vi "NI VeriStand - Get Item Property.vi"   [LabVIEW 2020, in "Custom Device API.lvlib"]
doc: "Returns the <B>Value</B> of a specific item <B>Property Name</B>. Properties do not inherit within a custom device, so <B>Item Ref in</B> must reference the specific item on which the property is set. \n\nFor instances with a <B>Default Value</B> input, the <B>Value</B> output returns this value if the <B>Property Name</B> is not found for the specified item. Wire data to the <B>Default Value</B> input to determine the polymorphic instance to use or manually select the instance."
uses:
  <vilib>/NI VeriStand/Custom Device API/Custom Device API.lvlib
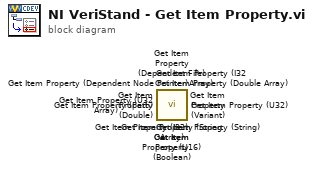
[diagram p0: block diagram]
diagram:
  n1 = call <vilib>:"Get Item Property (String Array).vi"() -> ()  [unwired: 8 in, 4 out]
  n2 = call <vilib>:"Get Item Property (I32 Array).vi"() -> ()  [unwired: 8 in, 4 out]
  n3 = call <vilib>:"Get Item Property (U32 Array).vi"() -> ()  [unwired: 8 in, 4 out]
  n4 = call <vilib>:"Get Item Property (U32).vi"() -> ()  [unwired: 8 in, 4 out]
  n5 = call <vilib>:"Get Item Property (Dependent Node Pointer).vi"() -> ()  [unwired: 8 in, 4 out]
  n6 = call <vilib>:"Get Item Property (Dependent File).vi"() -> ()  [unwired: 7 in, 5 out]
  n7 = call <vilib>:"Get Item Property (Variant).vi"() -> ()  [unwired: 8 in, 4 out]
  n8 = call <vilib>:"Get Item Property (U16).vi"() -> ()  [unwired: 8 in, 4 out]
  n9 = call <vilib>:"Get Item Property (String).vi"() -> ()  [unwired: 8 in, 4 out]
  n10 = call <vilib>:"Get Item Property (Path).vi"() -> ()  [unwired: 8 in, 4 out]
  n11 = call <vilib>:"Get Item Property (I32).vi"() -> ()  [unwired: 8 in, 4 out]
  n12 = call <vilib>:"Get Item Property (Double).vi"() -> ()  [unwired: 8 in, 4 out]
  n13 = call <vilib>:"Get Item Property (Double Array).vi"() -> ()  [unwired: 8 in, 4 out]
  n14 = call <vilib>:"Get Item Property (Boolean).vi"() -> ()  [unwired: 8 in, 4 out]
